vi "Duplicate_Request.vi"(0 "Enable":bool=TRUE, 2 "New Name":string, 5 "error in (no error)":errorcluster) -> (17 "New Name":string, 18 "OK":bool, 19 "error out":errorcluster)   [LabVIEW 2022 SP3]
doc: "Displays a standard dialog box that prompts users to enter information, such as a user name and password.\n--------------------\n\nThis Express VI is configured as follows:\n\nMessage to Display to the User:Please enter the new test name (the instrument name stays the same)\nThe inputs are: \nText Entry Box: New Name"
panel:
  out "String":string="Please enter the new test name (the instrument name stays the same)"
  in  "Cancel":bool
  in  "OK2":bool
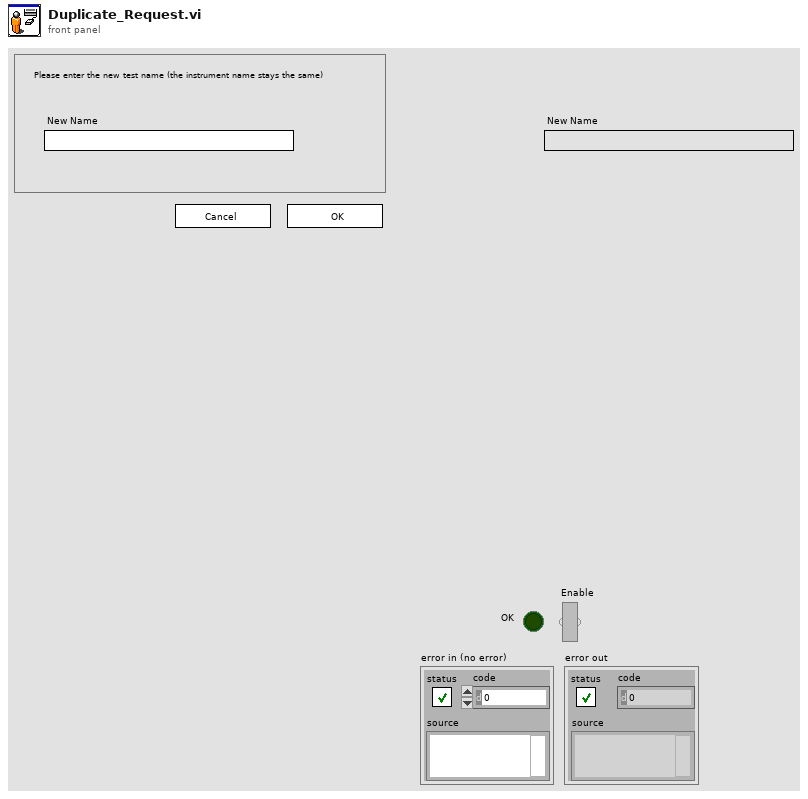
[diagram p1: front panel]
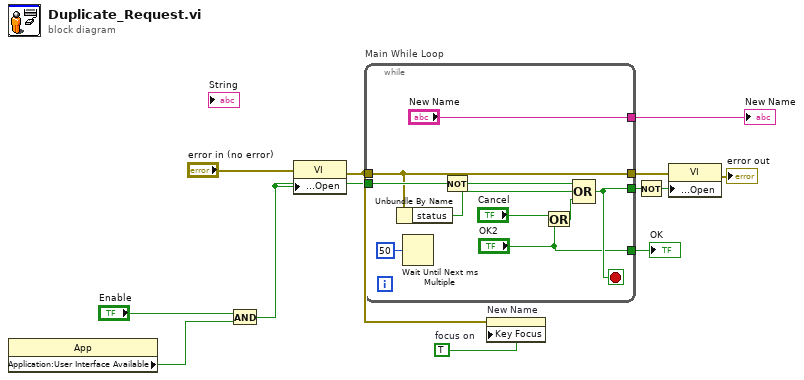
[diagram p0: block diagram]
diagram:
  w2 = TRUE  # focus on
  n1 = property class="App"() -> ("Application:User Interface Available"=w4:bool)  [unwired: 2 in, 2 out]
  n2 = And(x="Enable", y=w4) -> (x .and. y?=w5:bool)
  n3 = property class="VI"(error in="error in (no error)", "Front Panel Window:Open"=w5) -> (error out=w9:errorcluster)  [unwired: 1 in, 1 out]
  n4 = while "Main While Loop" {
    tunnel: ["OK2"] -> w12
    tunnel: w5 -> [w20]
    tunnel: [w18] -> w10
    tunnel: w9 -> [w17]
    tunnel: [w17] -> w8
    tunnel: ["New Name"] -> w3
    stop <- w18 stop-if-true
    n5 = Unbundle By Name(w17) -> ("status"=w15:bool)
    n6 = Wait Until Next ms Multiple(millisecond multiple=u32 50) -> ()  [unwired: 1 out]
    n7 = Not(x=w20) -> (.not. x?=w19:bool)
    n8 = Or(x="Cancel", y="OK2") -> (x .or. y?=w16:bool)
    n9 = Compound Arithmetic op=OR(w19, w15, w16) -> (w18:bool)
  }
  "OK" <- w12
  "New Name" <- w3
  n10 = property on="New Name" class="Str"(error in=w9, "Key Focus"=w2) -> ()  [unwired: 1 in, 2 out]
  n11 = Not(x=w10) -> (.not. x?=w11:bool)
  n12 = property class="VI"(error in=w8, "Front Panel Window:Open"=w11) -> (error out=→"error out":errorcluster)  [unwired: 1 in, 1 out]
